vi "Error Handler - Logging Message Loop.vi"(8 "error in (no error)":T1 caption="entrée d'erreur (pas d'erreur)", 10 "Erreurs à ignorer (exécution)":i32[](array[numeric]), 11 "File d'attente de messages":refnum<queue>) -> (0 "erreur en entrée dup.":T1, 3 "File d'attente de message dup.":refnum<queue>)   [LabVIEW 2018, in "Logging.lvlib"]
doc: "Traite une erreur qui a eu lieu dans la boucle de messages d'enregistrement en l'ignorant ou en générant un message \"Error\"."
uses:
  Logging.lvlib
  support/Message Queue/Message Cluster.ctl
  support/Message Queue/Message Queue.lvlib
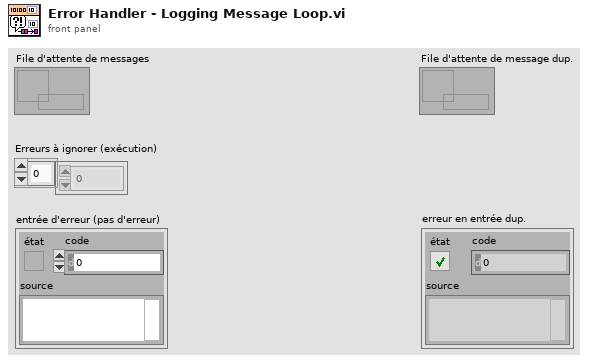
[diagram p1: front panel]
types:
  T1 = cluster{"état":bool, "code":i32, "source":string}
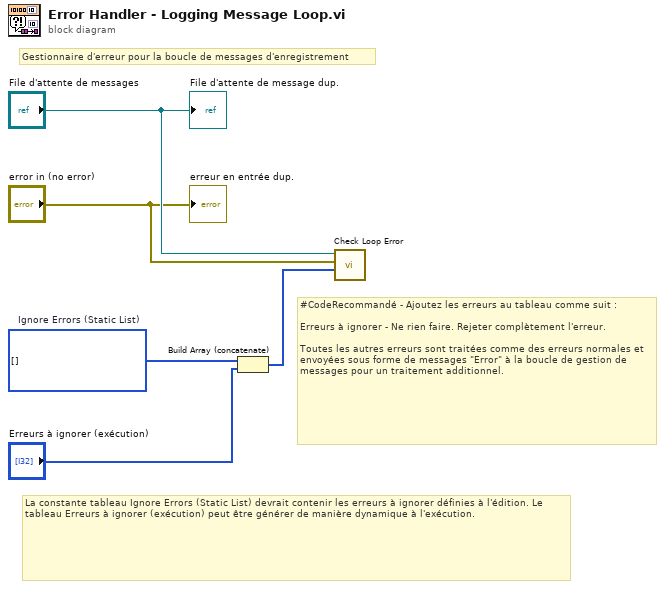
[diagram p0: block diagram]
diagram:
  w4 = i32[] []  # Ignore Errors (Static List)
  # "La constante tableau Ignore Errors (Static List) devrait contenir les erreurs à ignorer définies à l'édition. Le tableau Erreurs à ignorer (exécution) peut être générer de manière dynamique à l'exécution."
  # "#CodeRecommandé - Ajoutez les erreurs au tableau comme suit :\n\nErreurs à ignorer - Ne rien faire. Rejeter complètement l'erreur.\n\nToutes les autres erreurs sont traitées comme des erreurs normales et envoyées sous forme de messages \"Error\" à la boucle de gestion de messages pour un traitement additionnel."
  # "Gestionnaire d'erreur pour la boucle de messages d'enregistrement"
  n1 = Build Array (concatenate)(w4, "Erreurs à ignorer (exécution)") -> (w3:i32[])
  n2 = call "Check Loop Error.vi"("Ignorer les erreurs"=w3, "erreur à traiter"="error in (no error)", "File d'attente de messages"="File d'attente de messages") -> ()  [unwired: 7 in, 2 out]
  "File d'attente de message dup." <- "File d'attente de messages"
  "erreur en entrée dup." <- "error in (no error)"
